vi "WSVCAP SHL Host TL Tester.vi"() -> ()   [LabVIEW 2012]
uses:
  Type Defs/WSVCAP SHL DUT Number Enum.ctl
  <vilib>/userdefined/High Color/nirio_resource_hc.ctl
  Type Defs/WSVCAP SHL Tester System Cluster.ctl
  Type Defs/WSVCAP SHL I2C DUT Mask Mode Enum.ctl
panel:
  in  "C3 Cap DAC":u8=144 caption="B Data In" format="0x%02x"
  in  "C2 Cap DAC":u8=144 caption="B Data In" format="0x%02x"
  in  "C1 Cap DAC":u8=144 caption="B Data In" format="0x%02x"
  in  "Set Cap DAC":bool
  in  "CP 35V":bool
  in  "CP 23.75V":bool
  in  "DVA On":bool
  in  "DVA Off":bool
  in  "CP 44V":bool
  in  "CP 40.25V":bool
  in  "Read Data DUT CMD":string caption="Read Data Out"
  in  "Read DUT":bool
  in  "CP On":bool
  in  "CP Off":bool
  in  "Write DUT":bool
  in  "Write Data DUT":string caption="Write Data Out"
  out "Read Data DUT Out":string caption="Data In"
  in  "Stop RFFE Cycle":bool
  in  "Start RFFE Cycle":bool
  in  "Command":string[](array[string])=["0702013B3B3B", "070201000000"]
  in  "Post CMd Delay":dbl[](array[numeric])=[1.2e-05, 5.4e-05] min=0.0 max=0.5 format="%#.0p s"
  in  "Number of Commands":u32=2 min=1 max=4 step=1
  out "Cycle Count":u64=2 min=1 max=4 step=1
  in  "Monitor":bool
  out "AD7747 Values":string[][](table)
  in  "Mode":enum32{"C1", "C2", "C3", "All", "Single"}(radio)
  in  "RFFE Slave Address":u8=144 caption="Slave Address" format="0x%02x"
  out "Activity Log":string
  out "Simulate FPGA":bool
  out "Online":bool
  out "FPGA Resource":T1
  out "Status":string
  out "Busy":bool
  in  "I2C Bytes to Read":u8=1 caption="Bytes" min=1 max=4 step=1
  in  "Device":enum32{"C1", "C2", "C3"}(radio)
  in  "Exit":bool
  out "Read Data I2C":u8[](array[numeric]) caption="Data In" format="0x%02x"
  in  "Read Reg I2C":u8 caption="Register" format="0x%02x"
  in  "Read I2C":bool
  in  "DUT":T2
  in  "Write Data I2C":u8 caption="Data Out" format="0x%02x"
  in  "Write Reg I2C":u8=144 caption="Register" format="0x%02x"
  in  "I2C Init":bool
  in  "Init Data":u8[](array[numeric])=[164, 160, 14, 33] caption="Data Out" format="0x%02x"
  in  "Init Reg":u8[](array[numeric])=[191, 7, 9, 10] caption="Register" format="0x%02x"
  in  "Write I2C":bool
  in  "I2C Slave Address":u8=144 caption="Slave Address" format="0x%02x"
  in  "RFFE Clock Rate (Hz)":dbl=1000000.0 caption="Clock Rate" format="%.1p Hz"
  in  "I2C Clock Rate (Hz)":dbl=100000.0 caption="Clock Rate" format="%.0p Hz"
  in  "Error":errorcluster
  # "WS1050 Tester"
  # "AD7747 (I2C)"
  # "C1"
  # "C2"
  # "C3"
  # "DUT Control (RFFE)"
  # "DUT Cycling (RFFE)"
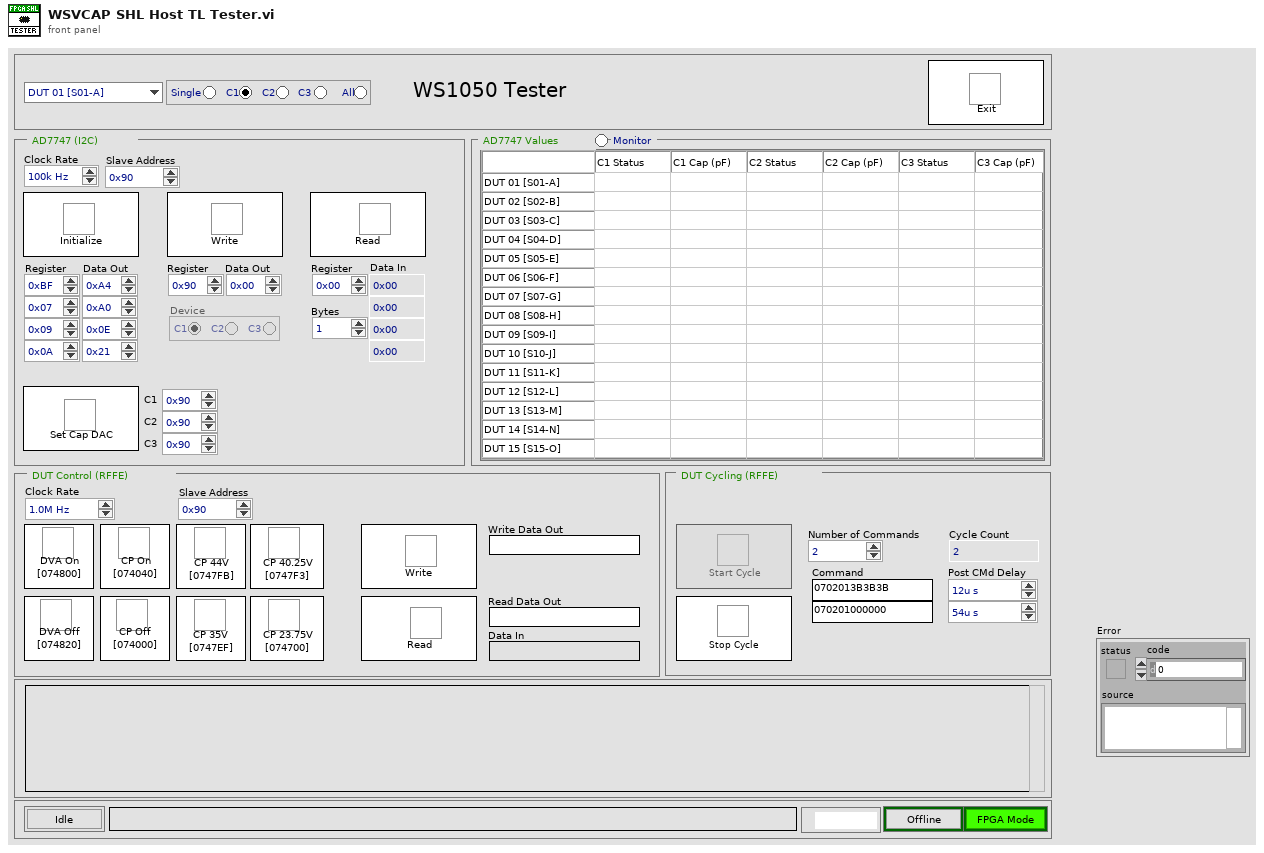
[diagram p1: front panel]
types:
  T1 = typedef "nirio_resource_hc.ctl" = tag
  T2 = typedef "WSVCAP SHL DUT Number Enum.ctl" = enum16{"DUT 01 [S01-A]", "DUT 02 [S02-B]", "DUT 03 [S03-C]", "DUT 04 [S04-D]", "DUT 05 [S05-E]", "DUT 06 [S06-F]", "DUT 07 [S07-G]", "DUT 08 [S08-H]", "DUT 09 [S09-I]", "DUT 10 [S10-J]", "DUT 11 [S11-K]", "DUT 12 [S12-L]", "DUT 13 [S13-M]", "DUT 14 [S14-N]", "DUT 15 [S15-O]", "DUT 16 [S16-P]"}
  T3 = typedef "WSVCAP SHL Tester System Cluster.ctl" = cluster{"I2C Monitor":bool, "SPI Cyle":bool, "SPI Mode":enum32{"Write/Read", "Cycle"}, "RFFE Cyle":bool, "RFFE Mode":enum32{"Write/Read", "Cycle"}}
  T4 = typedef "WSVCAP SHL Core System Cluster.ctl" = cluster{"Settings":T5, "FPGA Resource":tag, "Online":bool, "I2C Wait Ticks":u32, "SPI Wait Ticks":u32, "RFFE Wait Ticks":u32}
  T5 = typedef "WSVCAP SHL I2C Settings Cluster.ctl" = cluster{"FPGA Resource Name":string, "I2C Slave Address":u8, "I2C Clock Rate (Hz)":dbl, "SPI Clock Rate (Hz)":dbl, "RFFE Slave Address":u8, "RFFE Clock Rate (Hz)":dbl, "Simulate FPGA":bool, "C1 Cap DAC Default":u8, "C2 Cap DAC Default":u8, "C3 Cap DAC Default":u8}
  T6 = enum8{"Enabled", "Disabled", "Disabled and Grayed Out"}
  T7 = typedef "WSVCAP SHL I2C DUT Mask Mode Enum.ctl" = enum16{"Custom", "C1", "C2", "C3", "All"}
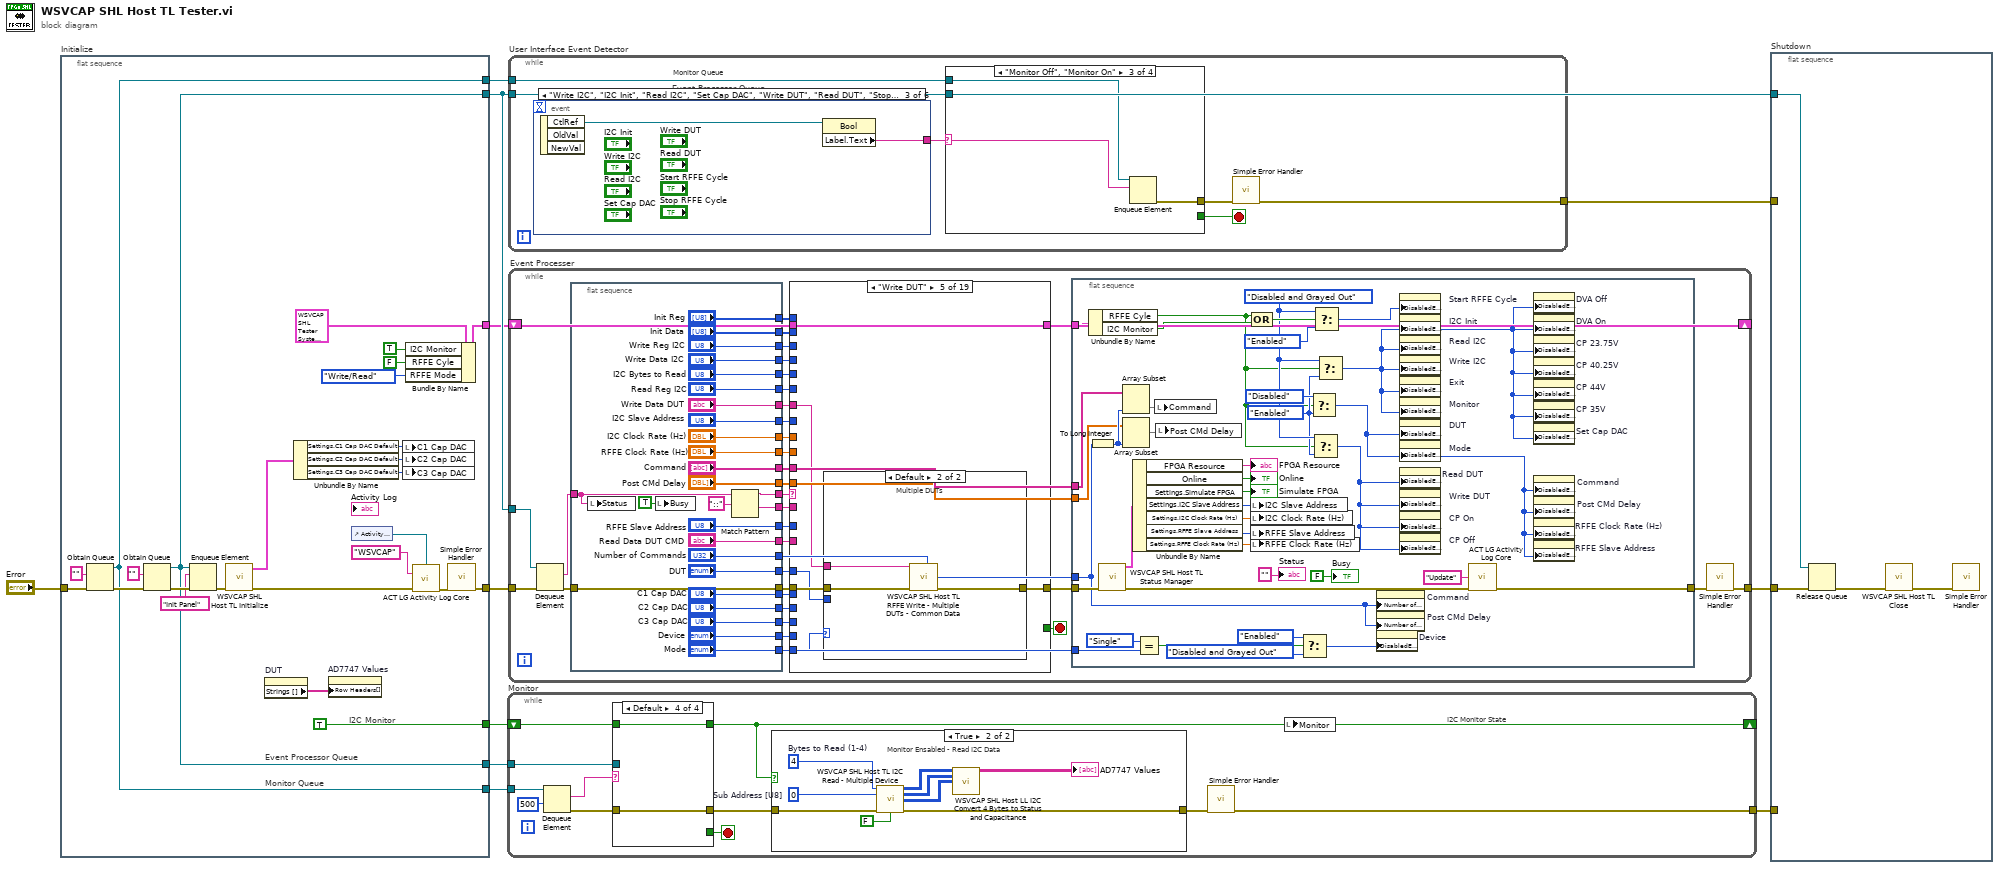
[diagram p0: block diagram]
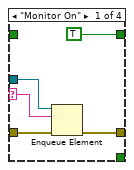
[diagram p2: hidden frame]
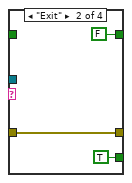
[diagram p3: hidden frame]
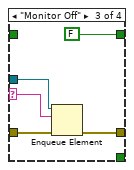
[diagram p4: hidden frame]
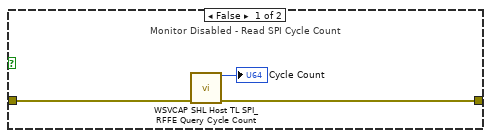
[diagram p5: hidden frame]
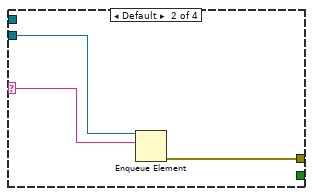
[diagram p7: hidden frame]
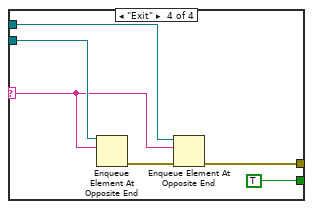
[diagram p8: hidden frame]
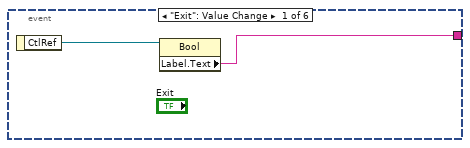
[diagram p9: hidden frame]
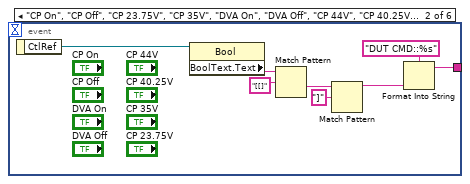
[diagram p10: hidden frame]
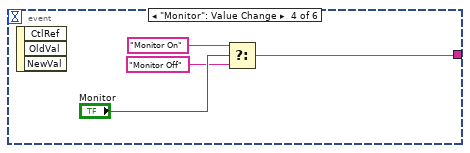
[diagram p11: hidden frame]
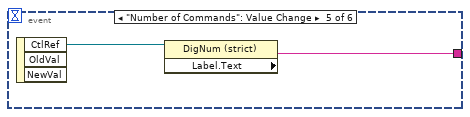
[diagram p12: hidden frame]
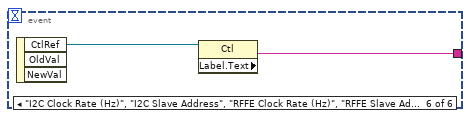
[diagram p13: hidden frame]
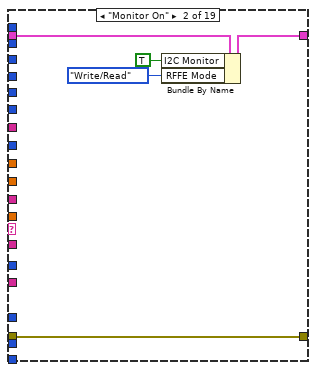
[diagram p15: hidden frame]
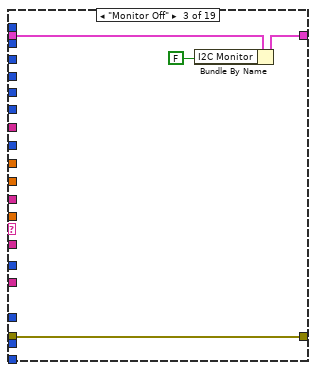
[diagram p16: hidden frame]
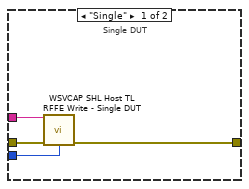
[diagram p18: hidden frame]
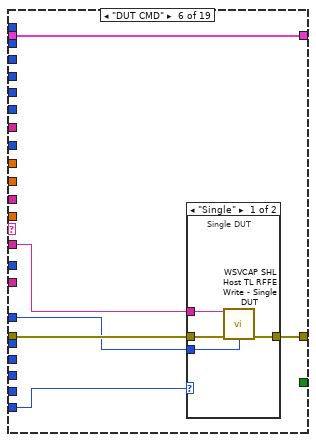
[diagram p19: hidden frame]
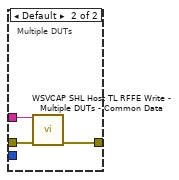
[diagram p20: hidden frame]
diagram:
  n1 = flat-sequence "Initialize" {
    tunnel: "Error" -> [w27]
    tunnel: [w25] -> w10
    tunnel: [TRUE ("Monitor")] -> w1
    tunnel: [w32] -> w6
    tunnel: [w23] -> w5
    tunnel: [w20] -> w4
    tunnel: [w25] -> w3
    tunnel: [w20] -> w2
    frame #0 {
      # "I2C Monitor"
      # "Monitor Queue"
      # "Event Processor Queue"
      n2 = Obtain Queue(element data type="" ("name (unnamed)"), error in (no error)=w27) -> (queue out=w20:refnum<queue>, error out=w26:errorcluster)  [unwired: 3 in, 1 out]
      n3 = Obtain Queue(element data type="" ("name (unnamed)"), error in (no error)=w26) -> (queue out=w25:refnum<queue>, error out=w35:errorcluster)  [unwired: 3 in, 1 out]
      n4 = Enqueue Element(queue=w25, element="Init Panel" ("name (unnamed)"), error in (no error)=w35) -> (error out=w17:errorcluster)  [unwired: 1 in, 2 out]
      n5 = call "WSVCAP SHL Host TL Initialize.vi"("error in"=w17) -> ("System"=w15:T4, "error out"=w16:errorcluster)  [unwired: 13 in]
      n6 = property on="DUT" class="Enum (strict)"() -> ("Strings []"=w18:string[])  [unwired: 2 in, 2 out]
      n7 = Unbundle By Name(w15) -> ("Settings.C1 Cap DAC Default"=w14:u8, "Settings.C2 Cap DAC Default"=w13:u8, "Settings.C3 Cap DAC Default"=w12:u8)
      n8 = property on="AD7747 Values" class="Tbl (strict)"("Row Headers[]"=w18) -> ()  [unwired: 2 in, 2 out]
      n9 = control-ref of="Activity Log"() -> (w31:refnum<vi>)
      n10 = local write "C1 Cap DAC"(w14) -> ()
      n11 = local write "C2 Cap DAC"(w13) -> ()
      n12 = local write "C3 Cap DAC"(w12) -> ()
      n13 = Bundle By Name(cluster=T3 {"I2C Monitor"=TRUE, "SPI Cyle"=TRUE, "SPI Mode"=enum."Write/Read", "RFFE Cyle"=FALSE, "RFFE Mode"=enum."Write/Read"}, "I2C Monitor"=TRUE, "RFFE Cyle"=FALSE ("I2C Monitor"), "RFFE Mode"=enum32{"Write/Read", "Cycle"}."Write/Read" ("SPI Mode")) -> (w23:T3)
      n14 = call "ACT LG Activity Log Core.vi"("Display Ref"=w31, "Source"="WSVCAP", "Error In (no error)"=w16) -> ("Error Out"=w33:errorcluster)  [unwired: 11 in, 1 out]
      n15 = call <vilib>:"Simple Error Handler.vi"("error in (no error)"=w33) -> ("error out"=w32:errorcluster)  [unwired: 4 in, 4 out]
    }
  }
  n16 = while "Monitor" {
    tunnel: [w38] -> w7
    shift-right: [w37] -> _
    shift-left: w1 -> [w44]
    tunnel: w4 -> [w42]
    tunnel: w3 -> [w41]
    stop <- w39 stop-if-true
    # "I2C Monitor State"
    n17 = Dequeue Element(queue=w42, timeout in ms (-1)=500 ("Wait Time (500ms)")) -> (element=w45:string, error out=w43:errorcluster)  [unwired: 1 in, 2 out]
    n18 = case shown="Default" w45 {
      selector: w45 -> [w49 _ w57 _]
      tunnel: [TRUE FALSE FALSE w62] -> w37
      tunnel: w44 -> [_ _ _ w62]
      tunnel: w43 -> [w51 w54 w59 w61]
      tunnel: [w50 w54 w58 w61] -> w40
      tunnel: w41 -> [w48 _ w56 _]
      tunnel: [_ TRUE _ _] -> w39
      frame "Monitor On" {
        n19 = Enqueue Element(queue=w48, element=w49, error in (no error)=w51) -> (error out=w50:errorcluster)  [unwired: 1 in, 2 out]
      }
      frame "Exit" {
      }
      frame "Monitor Off" {
        n20 = Enqueue Element(queue=w56, element=w57, error in (no error)=w59) -> (error out=w58:errorcluster)  [unwired: 1 in, 2 out]
      }
      frame Default {
      }
    }
    n21 = case shown="True" w37 {
      tunnel: [w63 w68] -> w47
      tunnel: w40 -> [w64 w69]
      frame False {
        # "Monitor Disabled - Read SPI Cycle Count"
        n22 = call "WSVCAP SHL Host TL SPI_RFFE Query Cycle Count.vi"("error in"=w64) -> ("Cycle Count"=→"Cycle Count":u64, "error out"=w63:errorcluster)  [unwired: 13 in]
      }
      frame True {
        w73 = u8 4  # Bytes to Read (1-4)
        w74 = u8 0  # Sub Address [U8]
        # "Monitor Ensabled - Read I2C Data"
        n23 = call "WSVCAP SHL Host TL I2C Read - Multiple Device.vi"("Bytes to Read (1-4)"=w73, "Sub Address [U8]"=w74, "error in"=w69, "Log (T)"=FALSE) -> ("C1:1-16 Read Data [U8]"=w72:u8[][], "C2:1-16 Read Data [U8]"=w71:u8[][], "C3:1-16 Read Data [U8]"=w67:u8[][], "error out"=w68:errorcluster)  [unwired: 8 in]
        n24 = call "WSVCAP SHL Host LL I2C Convert 4 Bytes to Status and Capacitance.vi"("C1:1-16 Read Data [U8]"=w72, "C2_1-16 Read Data [U8]"=w71, "C3_1-16 Read Data [U8]"=w67) -> ("AD7747 Values"=→"AD7747 Values":string[][])  [unwired: 12 in]
      }
    }
    n25 = call <vilib>:"Simple Error Handler.vi"("error in (no error)"=w47) -> ("error out"=w38:errorcluster)  [unwired: 4 in, 4 out]
    n26 = local write "Monitor"(w37) -> ()
  }
  n27 = while "User Interface Event Detector" {
    tunnel: w10 -> [w79]
    tunnel: [w76] -> w8
    tunnel: w2 -> [w75]
    stop <- w77 stop-if-true
    # "Monitor Queue"
    # "Event Processor Queue"
    n28 = event shown="[2] \"Write I2C\", \"I2C Init\", \"Read I2C\", \"Set Cap DAC\", \"Write DUT\", \"Read DUT\", \"Stop RFFE Cycle\", \"Start RFFE Cycle\": Value Change" {
      selector: _ -> [_ _ _ _ _ _]
      dyn-events: _ -> [_ _ _ _ _ _]
      timeout: _ -> [_ _ _ _ _ _]
      tunnel: [w93 w101 w104 w105 w110 w112] -> w80
      event "Exit": Value Change {
        n29 = event-data() -> ("CtlRef"=w94:refnum<vi>)  [unwired: 1 in]
        n30 = property class="Bool"(reference=w94) -> ("Label.Text"=w93:string)  [unwired: 1 in, 2 out]
      }
      event "CP On", "CP Off", "CP 23.75V", "CP 35V", "DVA On", "DVA Off", "CP 44V", "CP 40.25V": Value Change {
        n31 = event-data() -> ("CtlRef"=w102:refnum<vi>)  [unwired: 1 in]
        n32 = property class="Bool"(reference=w102) -> ("BoolText.Text"=w99:string)  [unwired: 1 in, 2 out]
        n33 = Match Pattern(string=w99, regular expression="[[]") -> (after substring=w97:string)  [unwired: 1 in, 3 out]
        n34 = Match Pattern(string=w97, regular expression="]") -> (before substring=w95:string)  [unwired: 1 in, 3 out]
        n35 = Format Into String(format string="DUT CMD::%s", w95) -> (resulting string=w101:string)  [unwired: 2 in, 1 out]
      }
      event "Write I2C", "I2C Init", "Read I2C", "Set Cap DAC", "Write DUT", "Read DUT", "Stop RFFE Cycle", "Start RFFE Cycle": Value Change {
        n36 = event-data() -> ("CtlRef"=w103:refnum<vi>)  [unwired: 1 in, 2 out]
        n37 = property class="Bool"(reference=w103) -> ("Label.Text"=w104:string)  [unwired: 1 in, 2 out]
      }
      event "Monitor": Value Change {
        n38 = event-data() -> ()  [unwired: 1 in, 3 out]
        n39 = Select(t="Monitor On" ("Label.Text"), s="Monitor", f="Monitor Off" ("Label.Text")) -> (s? t:f=w105:string)
      }
      event "Number of Commands": Value Change {
        n40 = event-data() -> ("CtlRef"=w109:refnum<vi>)  [unwired: 1 in, 2 out]
        n41 = property class="DigNum (strict)"(reference=w109) -> ("Label.Text"=w110:string)  [unwired: 1 in, 2 out]
      }
      event "I2C Clock Rate (Hz)", "I2C Slave Address", "RFFE Clock Rate (Hz)", "RFFE Slave Address", "Mode": Value Change {
        n42 = event-data() -> ("CtlRef"=w111:refnum<vi>)  [unwired: 1 in, 2 out]
        n43 = property class="Ctl"(reference=w111) -> ("Label.Text"=w112:string)  [unwired: 1 in, 2 out]
      }
    }
    n44 = case shown="\"Monitor Off\", \"Monitor On\"" w80 {
      selector: w80 -> [_ w83 w86 w87]
      tunnel: w79 -> [_ w82 _ w92]
      tunnel: [_ w81 w85 w89] -> w78
      tunnel: [_ _ _ TRUE] -> w77
      tunnel: w75 -> [_ _ w84 w88]
      frame "" {
      }
      frame Default {
        n45 = Enqueue Element(queue=w82, element=w83) -> (error out=w81:errorcluster)  [unwired: 2 in, 2 out]
      }
      frame "Monitor Off", "Monitor On" {
        n46 = Enqueue Element(queue=w84, element=w86) -> (error out=w85:errorcluster)  [unwired: 2 in, 2 out]
      }
      frame "Exit" {
        n47 = Enqueue Element At Opposite End(queue=w92, element=w87) -> (error out=w90:errorcluster)  [unwired: 2 in, 2 out]
        n48 = Enqueue Element At Opposite End(queue=w88, element=w87, error in (no error)=w90) -> (error out=w89:errorcluster)  [unwired: 1 in, 2 out]
      }
    }
    n49 = call <vilib>:"Simple Error Handler.vi"("error in (no error)"=w78) -> ("error out"=w76:errorcluster)  [unwired: 4 in, 4 out]
  }
  n50 = while "Event Processer" {
    tunnel: w10 -> [w146]
    tunnel: [w144] -> w9
    tunnel: w6 -> [w125]
    shift-right: [w120] -> _
    shift-left: w5 -> [w121]
    stop <- w145 stop-if-true
    n51 = Dequeue Element(queue=w146, error in (no error)=w125) -> (element=w142:string, error out=w140:errorcluster)  [unwired: 1 in, 2 out]
    n52 = flat-sequence {
      tunnel: ["I2C Clock Rate (Hz)"] -> w143
      tunnel: [w190] -> w141
      tunnel: w142 -> [w191]
      tunnel: [w210] -> w139
      tunnel: w140 -> [w210]
      tunnel: ["I2C Bytes to Read"] -> w138
      tunnel: ["I2C Slave Address"] -> w137
      tunnel: ["RFFE Clock Rate (Hz)"] -> w136
      tunnel: ["DUT"] -> w133
      tunnel: ["Init Data"] -> w132
      tunnel: ["Init Reg"] -> w131
      tunnel: ["Write Reg I2C"] -> w130
      tunnel: ["Write Data I2C"] -> w129
      tunnel: ["Read Reg I2C"] -> w128
      tunnel: ["Write Data DUT"] -> w127
      tunnel: ["Mode"] -> w117
      tunnel: ["Device"] -> w126
      tunnel: ["Command"] -> w123
      tunnel: ["Post CMd Delay"] -> w122
      tunnel: ["Number of Commands"] -> w124
      tunnel: ["RFFE Slave Address"] -> w119
      tunnel: ["Read Data DUT CMD"] -> w118
      tunnel: [w188] -> w116
      tunnel: ["C1 Cap DAC"] -> w115
      tunnel: ["C2 Cap DAC"] -> w114
      tunnel: ["C3 Cap DAC"] -> w113
      frame #0 {
        n53 = local write "Status"(w191) -> ()
        n54 = local write "Busy"(TRUE ("Busy")) -> ()
        n55 = Match Pattern(string=w191, regular expression="::") -> (before substring=w190:string, after substring=w188:string)  [unwired: 1 in, 2 out]
      }
    }
    n56 = case shown="\"Write DUT\"" w141 {
      tunnel: w139 -> [w213 w218 w222 w224 w230 w243 w256 w274 w290 w311 w325 w330 w338 w357 w371 w400 w402 w408 w413]
      tunnel: [w213 w218 w222 w224 w229 w242 w255 w273 w289 w310 w324 w329 w337 w356 w370 w394 w402 w405 w411] -> w135
      tunnel: [_ _ _ _ _ _ _ _ _ _ _ _ _ _ _ _ TRUE _ _] -> w145
      tunnel: w143 -> [_ _ _ _ _ _ _ _ _ _ _ _ _ _ _ _ _ w407 _]
      tunnel: w138 -> [_ _ _ _ _ _ _ _ _ _ _ _ _ _ _ w396 _ _ _]
      tunnel: w137 -> [_ _ _ _ _ _ _ _ _ _ _ _ _ _ _ _ _ w406 _]
      tunnel: w136 -> [_ _ _ _ _ _ _ _ _ _ _ _ _ _ _ _ _ _ w412]
      tunnel: w133 -> [_ _ _ _ w227 w240 w253 w271 w287 w308 _ _ w335 _ w368 w399 _ _ _]
      tunnel: w132 -> [_ _ _ _ _ _ _ _ _ _ _ _ _ _ w365 _ _ _ _]
      tunnel: w131 -> [_ _ _ _ _ _ _ _ _ _ _ _ _ _ w366 _ _ _ _]
      tunnel: w130 -> [_ _ _ _ _ _ _ _ _ _ _ _ w333 _ _ _ _ _ _]
      tunnel: w129 -> [_ _ _ _ _ _ _ _ _ _ _ _ w332 _ _ _ _ _ _]
      tunnel: w128 -> [_ _ _ _ _ _ _ _ _ _ _ _ _ _ _ w397 _ _ _]
      tunnel: w127 -> [_ _ _ _ w226 _ _ w270 _ _ _ _ _ _ _ _ _ _ _]
      tunnel: w117 -> [_ _ _ _ w228 w241 w254 w272 w288 w309 _ _ w336 _ w369 _ _ _ _]
      tunnel: w126 -> [_ _ _ _ _ _ _ _ _ _ _ _ w334 _ w367 w398 _ _ _]
      tunnel: w123 -> [_ _ _ _ _ _ _ _ w286 w307 _ _ _ _ _ _ _ _ _]
      tunnel: w122 -> [_ _ _ _ _ _ _ _ w285 w306 _ _ _ _ _ _ _ _ _]
      tunnel: [w212 w216 w220 w223 w225 w239 w252 w269 w283 w304 w321 w326 w331 w363 w364 w393 w401 w404 w410] -> w120
      tunnel: w121 -> [w212 w217 w221 w223 w225 w239 w252 w269 w284 w305 w322 w327 w331 w363 w364 w393 w401 w404 w410]
      tunnel: w119 -> [_ _ _ _ _ _ _ _ _ _ _ _ _ _ _ _ _ _ w409]
      tunnel: w118 -> [_ _ _ _ _ _ w251 _ _ _ _ _ _ _ _ _ _ _ _]
      tunnel: w116 -> [_ _ _ _ _ w238 _ _ _ _ _ _ _ _ _ _ _ _ _]
      tunnel: w115 -> [_ _ _ _ _ _ _ _ _ w302 _ _ _ w355 _ _ _ _ _]
      tunnel: w114 -> [_ _ _ _ _ _ _ _ _ w301 _ _ _ w354 _ _ _ _ _]
      tunnel: w113 -> [_ _ _ _ _ _ _ _ _ w300 _ _ _ w353 _ _ _ _ _]
      frame Default {
      }
      frame "Monitor On" {
        n57 = Bundle By Name(cluster=w217, "I2C Monitor"=TRUE, "RFFE Mode"=enum32{"Write/Read", "Cycle"}."Write/Read" ("SPI Mode")) -> (w216:T3)
      }
      frame "Monitor Off" {
        n58 = Bundle By Name(cluster=w221, "I2C Monitor"=FALSE) -> (w220:T3)
      }
      frame "Number of Commands" {
      }
      frame "Write DUT" {
        n59 = case shown="Default" w228 {
          tunnel: w230 -> [w234 w237]
          tunnel: [w231 w236] -> w229
          tunnel: w227 -> [w232 _]
          tunnel: w226 -> [w233 w235]
          frame "Single" {
            # "Single DUT"
            n60 = call "WSVCAP SHL Host TL RFFE Write - Single DUT.vi"("Data Out"=w233, "error in"=w234, "DUT"=w232) -> ("error out"=w231:errorcluster)  [unwired: 12 in]
          }
          frame Default {
            # "Multiple DUTs"
            n61 = call "WSVCAP SHL Host TL RFFE Write - Multiple DUTs - Common Data.vi"("Data Out"=w235, "error in"=w237) -> ("error out"=w236:errorcluster)  [unwired: 13 in]
          }
        }
      }
      frame "DUT CMD" {
        n62 = case shown="\"Single\"" w241 {
          tunnel: w243 -> [w247 w250]
          tunnel: [w244 w249] -> w242
          tunnel: w240 -> [w245 _]
          tunnel: w238 -> [w246 w248]
          frame "Single" {
            # "Single DUT"
            n63 = call "WSVCAP SHL Host TL RFFE Write - Single DUT.vi"("Data Out"=w246, "error in"=w247, "DUT"=w245) -> ("error out"=w244:errorcluster)  [unwired: 12 in]
          }
          frame Default {
            # "Multiple DUTs"
            n64 = call "WSVCAP SHL Host TL RFFE Write - Multiple DUTs - Common Data.vi"("Data Out"=w248, "error in"=w250) -> ("error out"=w249:errorcluster)  [unwired: 13 in]
          }
        }
      }
      frame "Read DUT" {
        n65 = case shown="Default" w254 {
          tunnel: w256 -> [w261 w268]
          tunnel: [w259 w267] -> w255
          tunnel: w253 -> [w260 w264]
          tunnel: w251 -> [w257 w266]
          frame "Single" {
            # "Single DUT"
            n66 = call "WSVCAP SHL Host TL RFFE Read - Single DUT.vi"("Data Out"=w257, "error in"=w261, "DUT"=w260) -> ("Data In"=→"Read Data DUT Out":string, "error out"=w259:errorcluster)  [unwired: 11 in]
          }
          frame Default {
            # "Multiple DUTs"
            n67 = To Long Integer(number=w264) -> (32bit integer=w263:i32)
            n68 = call "WSVCAP SHL Host TL RFFE Read - Multiple DUTs - Common Data.vi"("Data Out"=w266, "error in"=w268) -> ("RFFE Data In"=w265:string[], "error out"=w267:errorcluster)  [unwired: 12 in]
            n69 = Index Array(array=w265, index=w263) -> (element=w262:string)
            n70 = local write "Read Data DUT Out"(w262) -> ()
          }
        }
      }
      frame "Write/Read DUT" {
        n71 = case shown="\"C2\"" w272 {
          tunnel: w274 -> [w278 w281]
          tunnel: [w276 w280] -> w273
          tunnel: w271 -> [w277 _]
          tunnel: w270 -> [w275 w279]
          frame "C1", Default {
            # "Single DUT"
            n72 = call "WSVCAP SHL Host TL SPI Write_Read - Single DUT.vi"("Data Out"=w275, "error in"=w278, "DUT"=w277) -> ("error out"=w276:errorcluster)  [unwired: 11 in, 1 out]
          }
          frame "C2" {
            # "Multiple DUTs"
            n73 = call "WSVCAP SHL Host TL SPI Write_Read - Multiple DUTs - Common Data.vi"("Data Out"=w279, "error in"=w281) -> ("error out"=w280:errorcluster)  [unwired: 12 in, 1 out]
          }
        }
      }
      frame "Start SPI Cycle" {
        n74 = case shown="\"C2\"" w288 {
          tunnel: w290 -> [w295 w299]
          tunnel: [w294 w298] -> w289
          tunnel: w287 -> [w293 _]
          tunnel: w286 -> [w292 w297]
          tunnel: w285 -> [w291 w296]
          frame "C1", Default {
            # "Single DUT"
            n75 = call "WSVCAP SHL Host TL SPI Write Cycle - Single DUT.vi"("Data Out (Cycle Commands)"=w292, "Post Command Delay"=w291, "error in"=w295, "DUT"=w293) -> ("error out"=w294:errorcluster)  [unwired: 11 in]
          }
          frame "C2" {
            # "Multiple DUTs"
            n76 = call "WSVCAP SHL Host TL SPI Write Cycle - Multiple DUTs - Common Data.vi"("Data Out (Cycle Commands)"=w297, "Post Command Delay"=w296, "error in"=w299) -> ("error out"=w298:errorcluster)  [unwired: 12 in]
          }
        }
        n77 = Bundle By Name(cluster=w284, "SPI Cyle"=TRUE) -> (w283:T3)
      }
      frame "Start RFFE Cycle" {
        n78 = case shown="\"All\"" w309 {
          tunnel: w311 -> [w316 w320]
          tunnel: [w315 w319] -> w310
          tunnel: w308 -> [w314 _]
          tunnel: w307 -> [w313 w318]
          tunnel: w306 -> [w312 w317]
          tunnel: w302 -> [_ _]
          tunnel: w301 -> [_ _]
          tunnel: w300 -> [_ _]
          frame Default {
            # "Single DUT"
            n79 = call "WSVCAP SHL Host TL RFFE Write Cycle - Single DUT.vi"("Data Out (Cycle Commands)"=w313, "Post Command Delay"=w312, "error in"=w316, "DUT"=w314) -> ("error out"=w315:errorcluster)  [unwired: 11 in]
          }
          frame "All" {
            # "Multiple DUTs"
            n80 = call "WSVCAP SHL Host TL RFFE Write Cycle - Multiple DUTs - Common Data.vi"("Data Out (Cycle Commands)"=w318, "Post Command Delay"=w317, "error in"=w320) -> ("error out"=w319:errorcluster)  [unwired: 12 in]
          }
        }
        n81 = Bundle By Name(cluster=w305, "RFFE Cyle"=TRUE ("SPI Cyle")) -> (w304:T3)
      }
      frame "Stop RFFE Cycle" {
        n82 = call "WSVCAP SHL Host TL RFFE Stop Write Cycle.vi"("error in"=w325) -> ("error out"=w324:errorcluster)  [unwired: 14 in]
        n83 = Bundle By Name(cluster=w322, "RFFE Cyle"=FALSE ("SPI Cyle")) -> (w321:T3)
      }
      frame "Stop SPI Cycle" {
        n84 = call "WSVCAP SHL Host TL SPI Stop Write Cycle.vi"("error in"=w330) -> ("error out"=w329:errorcluster)  [unwired: 14 in]
        n85 = Bundle By Name(cluster=w327, "SPI Cyle"=FALSE) -> (w326:T3)
      }
      frame "Write I2C" {
        n86 = case shown="\"Single\"" w336 {
          selector: w336 -> [_ w348]
          tunnel: w338 -> [w344 w352]
          tunnel: [w343 w351] -> w337
          tunnel: w335 -> [w341 _]
          tunnel: w333 -> [w340 w350]
          tunnel: w334 -> [w342 _]
          tunnel: w332 -> [w339 w349]
          frame "Single" {
            # "Single DUT"
            n87 = call "WSVCAP SHL Host TL I2C Write - Single Device.vi"("Sub Address [U8]"=w340, "Data Out [U8]"=w339, "error in"=w344, "DUT"=w341, "Device"=w342) -> ("error out"=w343:errorcluster)  [unwired: 10 in]
          }
          frame Default {
            # "Multiple DUTs"
            n88 = Format Into String(w348) -> (resulting string=w347:string)  [unwired: 3 in, 1 out]
            n89 = Scan From String(input string=w347, default 1=WSVCAP_SHL_I2C_DUT_Mask_Mode_Enum."All" ("DUT Mask Mode (All)")) -> (output 1=w345:T7)  [unwired: 3 in, 3 out]
            n90 = call "WSVCAP SHL Host TL I2C Write - Multiple Device - Common Data.vi"("Sub Address"=w350, "Data Out [U8]"=w349, "error in"=w352, "DUT Mask Mode (All)"=w345) -> ("error out"=w351:errorcluster)  [unwired: 11 in]
          }
        }
      }
      frame "Set Cap DAC" {
        w362 = 16 ("dimension size")
        n91 = Initialize Array(w355, w362) -> (w361:u8[])
        n92 = Initialize Array(w354, w362) -> (w360:u8[])
        n93 = Initialize Array(w353, w362) -> (w359:u8[])
        n94 = call "WSVCAP SHL Host TL I2C Write - Multiple Device - Unique Data.vi"("C1 Data"=w361, "C2 Data"=w360, "C3 Data"=w359, "Sub Address"=u8 11, "error in"=w357) -> ("error out"=w356:errorcluster)  [unwired: 10 in]
      }
      frame "I2C Init" {
        n95 = for {
          tunnel: w369 -> [w376]
          tunnel: w368 -> [w375]
          tunnel: w367 -> [w374]
          tunnel: w366 -> [w373] mode=indexing
          tunnel: w365 -> [w372] mode=indexing
          shift-right: [w377] -> w370
          shift-left: w371 -> [w378]
          n96 = case shown="Default" w376 {
            selector: w376 -> [_ w386]
            tunnel: w378 -> [w384 w392]
            tunnel: [w383 w391] -> w377
            tunnel: w375 -> [w381 _]
            tunnel: w374 -> [w382 _]
            tunnel: w373 -> [w380 w390]
            tunnel: w372 -> [w379 w389]
            frame "Single" {
              # "Single DUT"
              n97 = call "WSVCAP SHL Host TL I2C Write - Single Device.vi"("Sub Address [U8]"=w380, "Data Out [U8]"=w379, "error in"=w384, "DUT"=w381, "Device"=w382) -> ("error out"=w383:errorcluster)  [unwired: 10 in]
            }
            frame Default {
              # "Multiple DUTs"
              n98 = Format Into String(w386) -> (resulting string=w388:string)  [unwired: 3 in, 1 out]
              n99 = Scan From String(input string=w388, default 1=WSVCAP_SHL_I2C_DUT_Mask_Mode_Enum."All" ("DUT Mask Mode (All)")) -> (output 1=w385:T7)  [unwired: 3 in, 3 out]
              n100 = call "WSVCAP SHL Host TL I2C Write - Multiple Device - Common Data.vi"("Sub Address"=w390, "Data Out [U8]"=w389, "error in"=w392, "DUT Mask Mode (All)"=w385) -> ("error out"=w391:errorcluster)  [unwired: 11 in]
            }
          }
        }
      }
      frame "Read I2C" {
        n101 = call "WSVCAP SHL Host TL I2C Read - Single Device.vi"("Bytes to Read (1-4)"=w396, "Sub Address [U8]"=w397, "error in"=w400, "DUT"=w399, "Device"=w398) -> ("Device Data"=→"Read Data I2C":u8[], "error out"=w394:errorcluster)  [unwired: 9 in]
      }
      frame "Exit" {
      }
      frame "I2C Clock Rate (Hz)", "I2C Slave Address" {
        n102 = call "WSVCAP SHL Host TL I2C Configure.vi"("I2C_Slave Address"=w406, "Clock Rate (Hz)"=w407, "error in"=w408) -> ("error out"=w405:errorcluster)  [unwired: 11 in, 1 out]
      }
      frame "RFFE Clock Rate (Hz)", "RFFE Slave Address" {
        n103 = call "WSVCAP SHL Host TL RFFE Configure.vi"("RFFE Slave Address"=w409, "Clock Rate (Hz)"=w412, "error in"=w413) -> ("error out"=w411:errorcluster)  [unwired: 11 in, 1 out]
      }
    }
    n104 = flat-sequence {
      tunnel: [w172] -> w134
      tunnel: w135 -> [w182]
      tunnel: w124 -> [w171]
      tunnel: w123 -> [w169]
      tunnel: w122 -> [w167]
      tunnel: w120 -> [w165]
      tunnel: w117 -> [w155]
      frame #0 {
        w159 = T6."Enabled" ("Disabled")
        w160 = T6."Disabled and Grayed Out" ("Disabled")
        n105 = Unbundle By Name(w165) -> ("RFFE Cyle"=w158:bool, "I2C Monitor"=w164:bool)
        n106 = To Long Integer(number=w171) -> (32bit integer=w170:i32)
        n107 = call "WSVCAP SHL Host TL Status Manager.vi"("error in"=w182) -> ("System Out"=w181:T4, "error out"=w174:errorcluster)  [unwired: 13 in]
        n108 = Array Subset(array=w169, length=w170) -> (w168:string[])  [unwired: 1 in]
        n109 = Array Subset(array=w167, length=w170) -> (w166:dbl[])  [unwired: 1 in]
        n110 = Unbundle By Name(w181) -> ("FPGA Resource"=→"FPGA Resource":tag, "Online"=→"Online":bool, "Settings.Simulate FPGA"=→"Simulate FPGA":bool, "Settings.I2C Slave Address"=w180:u8, "Settings.I2C Clock Rate (Hz)"=w179:dbl, "Settings.RFFE Slave Address"=w156:u8, "Settings.RFFE Clock Rate (Hz)"=w178:dbl)
        n111 = Equal?(x=enum32{"C1", "C2", "C3", "All", "Single"}."Single" ("Mode"), y=w155) -> (x = y?=w151:bool)
        n112 = local write "Command"(w168) -> ()
        n113 = local write "Post CMd Delay"(w166) -> ()
        n114 = local write "I2C Slave Address"(w180) -> ()
        n115 = local write "I2C Clock Rate (Hz)"(w179) -> ()
        n116 = local write "RFFE Slave Address"(w156) -> ()
        n117 = local write "RFFE Clock Rate (Hz)"(w178) -> ()
        n118 = Compound Arithmetic op=OR(w158, w164) -> (w161:bool)
        n119 = Select(t=T6."Enabled" ("Disabled"), s=w151, f=T6."Disabled and Grayed Out" ("Disabled")) -> (s? t:f=w150:T6)
        n120 = Select(t=T6."Disabled" ("Disabled"), s=w158, f=w159) -> (s? t:f=w149:T6)
        n121 = Select(t=w160, s=w158, f=w159) -> (s? t:f=w147:T6)
        n122 = Select(t=w160, s=w161, f=T6."Enabled" ("Disabled")) -> (s? t:f=w157:T6)
        n123 = Select(t=w160, s=w158, f=w159) -> (s? t:f=w148:T6)
        n124 = property on="Command" class="Arr (strict)"("Number of Rows"=w171) -> ()  [unwired: 2 in, 2 out]
        n125 = property on="Post CMd Delay" class="Arr (strict)"("Number of Rows"=w171) -> ()  [unwired: 2 in, 2 out]
        n126 = property on="Device" class="RadioBtnsControl (strict)"("DisabledEnum"=w150) -> ()  [unwired: 2 in, 2 out]
        n127 = property on="Start RFFE Cycle" class="Bool"("DisabledEnum"=w157) -> ()  [unwired: 2 in, 2 out]
        n128 = property on="I2C Init" class="Bool"("DisabledEnum"=w148) -> ()  [unwired: 2 in, 2 out]
        n129 = property on="Read I2C" class="Bool"("DisabledEnum"=w148) -> ()  [unwired: 2 in, 2 out]
        n130 = property on="Write I2C" class="Bool"("DisabledEnum"=w148) -> ()  [unwired: 2 in, 2 out]
        n131 = property on="Exit" class="Bool"("DisabledEnum"=w148) -> ()  [unwired: 2 in, 2 out]
        n132 = property on="Monitor" class="Bool (strict)"("DisabledEnum"=w148) -> ()  [unwired: 2 in, 2 out]
        n133 = property on="DUT" class="Enum (strict)"("DisabledEnum"=w149) -> ()  [unwired: 2 in, 2 out]
        n134 = property on="Mode" class="RadioBtnsControl (strict)"("DisabledEnum"=w149) -> ()  [unwired: 2 in, 2 out]
        n135 = property on="Read DUT" class="Bool"("DisabledEnum"=w147) -> ()  [unwired: 2 in, 2 out]
        n136 = property on="Write DUT" class="Bool"("DisabledEnum"=w147) -> ()  [unwired: 2 in, 2 out]
        n137 = property on="CP On" class="Bool"("DisabledEnum"=w147) -> ()  [unwired: 2 in, 2 out]
        n138 = property on="CP Off" class="Bool"("DisabledEnum"=w147) -> ()  [unwired: 2 in, 2 out]
        n139 = call "ACT LG Activity Log Core.vi"("Log Line"="Update", "Error In (no error)"=w174) -> ("Error Out"=w172:errorcluster)  [unwired: 12 in, 1 out]
        n140 = property on="DVA Off" class="Bool"("DisabledEnum"=w148) -> ()  [unwired: 2 in, 2 out]
        n141 = property on="DVA On" class="Bool"("DisabledEnum"=w148) -> ()  [unwired: 2 in, 2 out]
        n142 = property on="CP 23.75V" class="Bool"("DisabledEnum"=w148) -> ()  [unwired: 2 in, 2 out]
        n143 = property on="CP 40.25V" class="Bool"("DisabledEnum"=w148) -> ()  [unwired: 2 in, 2 out]
        n144 = property on="CP 44V" class="Bool"("DisabledEnum"=w148) -> ()  [unwired: 2 in, 2 out]
        n145 = property on="CP 35V" class="Bool"("DisabledEnum"=w148) -> ()  [unwired: 2 in, 2 out]
        n146 = property on="Set Cap DAC" class="Bool"("DisabledEnum"=w148) -> ()  [unwired: 2 in, 2 out]
        n147 = property on="Command" class="Arr (strict)"("DisabledEnum"=w149) -> ()  [unwired: 2 in, 2 out]
        n148 = property on="Post CMd Delay" class="Arr (strict)"("DisabledEnum"=w149) -> ()  [unwired: 2 in, 2 out]
        n149 = property on="RFFE Clock Rate (Hz)" class="DigNum (strict)"("DisabledEnum"=w149) -> ()  [unwired: 2 in, 2 out]
        n150 = property on="RFFE Slave Address" class="DigNum (strict)"("DisabledEnum"=w149) -> ()  [unwired: 2 in, 2 out]
        "Busy" <- FALSE ("Busy")
        "Status" <- "" ("Status")
      }
    }
    n151 = call <vilib>:"Simple Error Handler.vi"("error in (no error)"=w134) -> ("error out"=w144:errorcluster)  [unwired: 4 in, 4 out]
  }
  n152 = flat-sequence "Shutdown" {
    tunnel: w10 -> [w417]
    tunnel: w9 -> [w416]
    tunnel: w8 -> [_]
    tunnel: w7 -> [_]
    frame #0 {
      n153 = Release Queue(queue=w417, error in (no error)=w416) -> (error out=w415:errorcluster)  [unwired: 1 in, 2 out]
      n154 = call "WSVCAP SHL Host TL Close.vi"("error in"=w415) -> ("error out"=w414:errorcluster)  [unwired: 14 in]
      n155 = call <vilib>:"Simple Error Handler.vi"("error in (no error)"=w414) -> ()  [unwired: 4 in, 5 out]
    }
  }
